vi "Read Configuration Parameters.vi"(8 "error in (no error)":errorcluster, 10 "refnum":T1, 11 "DispSnsr Configuration Dialog in":refnum<class "DispSnsr Configuration.lvclass">) -> (0 "error out":errorcluster, 2 "refnum out":T1, 3 "DispSnsr Configuration Dialog out":refnum<class "DispSnsr Configuration.lvclass">)   [LabVIEW 2016, in "Hardware.lvlib" / "Displacement Sensor.lvlib" / "DispSnsr Configuration.lvclass"]
uses:
  <userlib>/Common Components/Hardware/Displacement Sensor/DispSnsr Config/DispSnsr Configuration.lvclass
  <userlib>/Configuration Dialog Actor/Configuration.lvclass
  <vilib>/Utility/config.llb/NI_LVConfig.lvlib
  <userlib>/Common Components/Hardware/DevInfo/DevInfo.lvclass
  <userlib>/Common Components/Hardware/Displacement Sensor/DispSnsr/DispSnsr.lvclass
  <vilib>/Utility/config.llb/Config Data RefNum.ctl
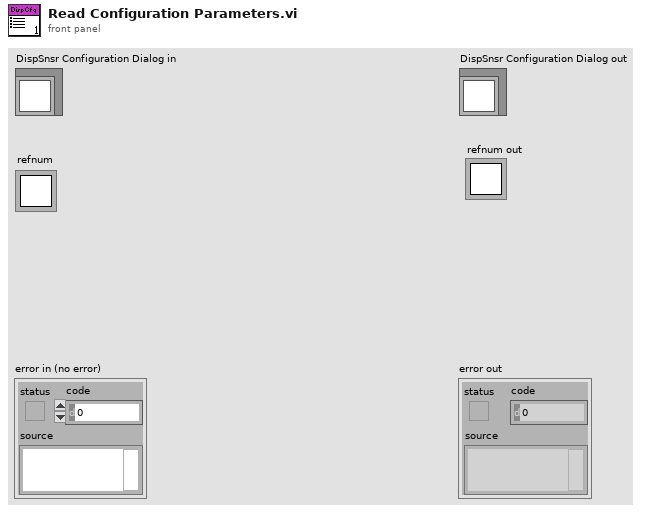
[diagram p1: front panel]
types:
  T1 = typedef "NI_LVConfig.lvlib/Config Data RefNum.ctl" = refnum<k1>
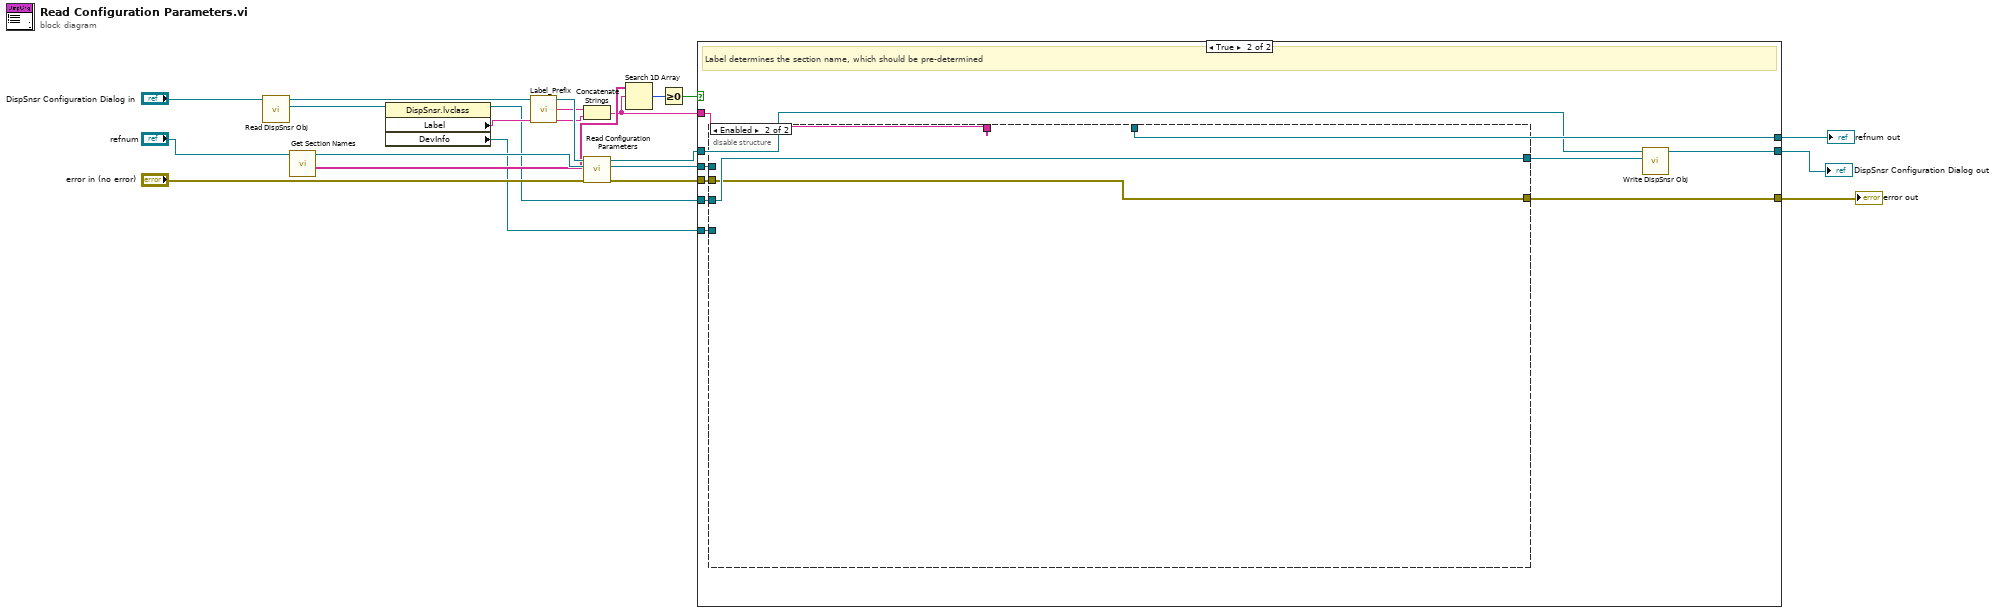
[diagram p0: block diagram]
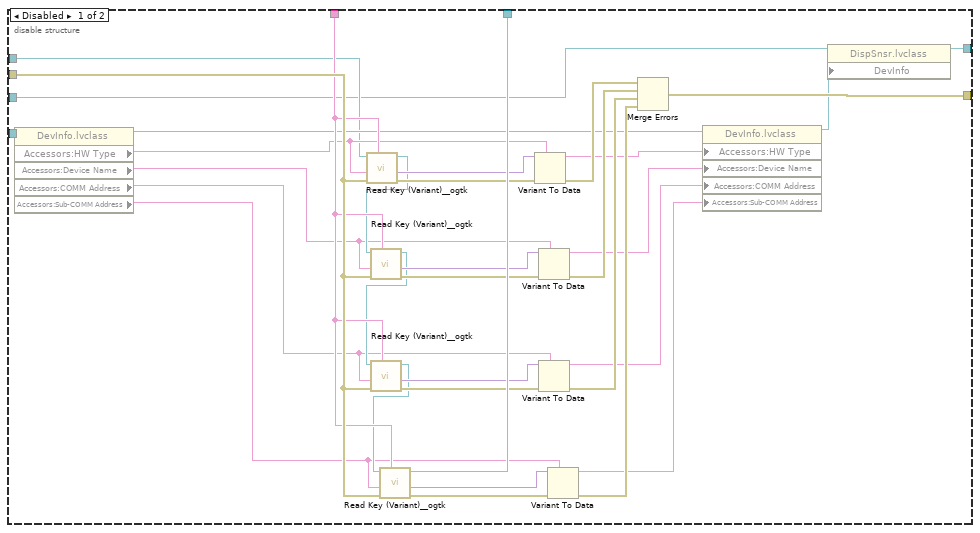
[diagram p3: hidden frame]
diagram:
  n1 = call <userlib>:"Read DispSnsr Obj.vi"("DispSnsr Configuration in"="DispSnsr Configuration Dialog in") -> ("Hardware.lvlib:Displacement Sensor.lvlib:DispSnsr.lvclass"=w9:refnum<class "DispSnsr.lvclass">, "DispSnsr Configuration out"=w11:refnum<class "DispSnsr Configuration.lvclass">)  [unwired: 9 in]
  n2 = call <vilib>:"Get Section Names.vi"("refnum"="refnum") -> ("section names"=w7:string[], "refnum out"=w8:T1)  [unwired: 8 in, 1 out]
  n3 = property class="DispSnsr.lvclass"(reference=w9) -> (reference out=w2:refnum<class "DispSnsr.lvclass">, "Label"=w3:string, "DevInfo"=w1:refnum<class "DevInfo.lvclass">)  [unwired: 1 in, 1 out]
  n4 = call <userlib>:"Label_Prefix.vi"() -> ("Label Prefix String"=w10:string)
  n5 = Concatenate Strings(w10, w3) -> (w6:string)
  n6 = call-parent "Read Configuration Parameters.vi"("error in (no error)"="error in (no error)", "refnum"=w8, "Configuration in"=w11) -> ("error out"=w17:errorcluster, "refnum out"=w18:T1, "Configuration out"=w16:refnum<class "DispSnsr Configuration.lvclass">)  [unwired: 6 in]
  n7 = Search 1D Array(1D array=w7, element=w6) -> (index of element=w5:i32)  [unwired: 1 in]
  n8 = Greater Or Equal To 0?(x=w5) -> (x >= 0?=w4:bool)
  n9 = case shown="True" w4 {
    tunnel: w18 -> [w22 w26]
    tunnel: w17 -> [w21 w33]
    tunnel: w16 -> [w23 w27]
    tunnel: [w23 w28] -> w15
    tunnel: [w22 w31] -> w14
    tunnel: [w21 w30] -> w13
    tunnel: w6 -> [_ w32]
    tunnel: w2 -> [_ w25]
    tunnel: w1 -> [_ w29]
    frame False {
    }
    frame True {
      # "Label determines the section name, which should be pre-determined"
      n10 = disable-structure shown="Enabled" {
        disable-tunnel: w33 -> [w66 w67]
        disable-tunnel: w32 -> [w65 _]
        disable-tunnel: [w64 _] -> w31
        disable-tunnel: [w63 w67] -> w30
        disable-tunnel: w29 -> [w47 _]
        disable-tunnel: [w36 w68] -> w24
        disable-tunnel: w26 -> [w35 _]
        disable-tunnel: w25 -> [w34 w68]
        frame Disabled {
          n11 = property class="DevInfo.lvclass"(reference=w47) -> (reference out=w42:refnum<class "DevInfo.lvclass">, "Accessors:HW Type"=w46:string, "Accessors:Device Name"=w45:string, "Accessors:COMM Address"=w44:string, "Accessors:Sub-COMM Address"=w43:string)  [unwired: 1 in, 1 out]
          n12 = call <userlib>:"Read Key (Variant)__ogtk.vi"("section"=w65, "error in (no error)"=w66, "type"=w46, "refnum"=w35) -> ("error out"=w61:errorcluster, "key-value"=w62:variant, "refnum out"=w54:T1)  [unwired: 4 in, 1 out]
          n13 = call <userlib>:"Read Key (Variant)__ogtk.vi"("section"=w65, "error in (no error)"=w66, "type"=w45, "refnum"=w54) -> ("error out"=w59:errorcluster, "key-value"=w60:variant, "refnum out"=w53:T1)  [unwired: 4 in, 1 out]
          n14 = call <userlib>:"Read Key (Variant)__ogtk.vi"("section"=w65, "error in (no error)"=w66, "type"=w44, "refnum"=w53) -> ("error out"=w57:errorcluster, "key-value"=w58:variant, "refnum out"=w52:T1)  [unwired: 4 in, 1 out]
          n15 = call <userlib>:"Read Key (Variant)__ogtk.vi"("section"=w65, "error in (no error)"=w66, "type"=w43, "refnum"=w52) -> ("error out"=w55:errorcluster, "key-value"=w56:variant, "refnum out"=w64:T1)  [unwired: 4 in, 1 out]
          n16 = Variant To Data(error in=w61, type=w46, Variant=w62) -> (data=w41:string, error out=w51:errorcluster)
          n17 = Variant To Data(error in=w59, type=w45, Variant=w60) -> (data=w40:string, error out=w50:errorcluster)
          n18 = Variant To Data(error in=w57, type=w44, Variant=w58) -> (data=w39:string, error out=w49:errorcluster)
          n19 = Variant To Data(error in=w55, type=w43, Variant=w56) -> (data=w38:string, error out=w48:errorcluster)
          n20 = Merge Errors(w51, w50, w49, w48) -> (w63:errorcluster)
          n21 = property class="DevInfo.lvclass"(reference=w42, "Accessors:HW Type"=w41, "Accessors:Device Name"=w40, "Accessors:COMM Address"=w39, "Accessors:Sub-COMM Address"=w38) -> (reference out=w37:refnum<class "DevInfo.lvclass">)  [unwired: 1 in, 1 out]
          n22 = property class="DispSnsr.lvclass"(reference=w34, "DevInfo"=w37) -> (reference out=w36:refnum<class "DispSnsr.lvclass">)  [unwired: 1 in, 1 out]
        }
        frame Enabled {
        }
      }
      n23 = call <userlib>:"Write DispSnsr Obj.vi"("Hardware.lvlib:Displacement Sensor.lvlib:DispSnsr.lvclass"=w24, "DispSnsr Configuration in"=w27) -> ("DispSnsr Configuration out"=w28:refnum<class "DispSnsr Configuration.lvclass">)  [unwired: 9 in]
    }
  }
  "DispSnsr Configuration Dialog out" <- w15
  "error out" <- w13
  "refnum out" <- w14
